vi "SMSMagnet.Contents.vi"   [LabVIEW 2014, in "SMSMagnet.lvlib"]
doc: "This is the constructor of a class.\n\nLicense Agreement for this software:\n\nCopyright (C)\nGesellschaft für Schwerionenforschung, GSI\nPlanckstr. 1\n64291 Darmstadt\nGermany\n\nContact: D.Beck@gsi.de \n\nThis program is free software; you can redistribute it and/or modify it under the terms of the \nGNU General Public License as published by the Free Software Foundation; either version 2 of \nthe license, or (at your option) any later version.\n\nThis program is distributed in the hope that it will be useful, but WITHOUT ANY WARRANTY; \nwithout even the implied warranty of MERCHANTABILITY or FITNESS FOR A PARTICULAR PURPOSE. See the GNU General License for more details (http://www.gnu.org).\n\nGesellschaft für Schwerionenforschung, GSI\nPlanckstr. 1, 64291 Darmstadt, Germany\nFor all questions and ideas contact: M.Richter@gsi.de, H.Brand@gsi.de or D.Beck@gsi.de.\nLast update: 16-JUN-2004"
uses:
  SMSMagnet.lvlib
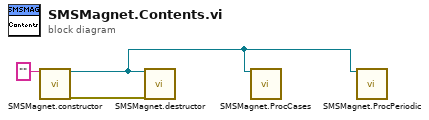
[diagram p0: block diagram]
diagram:
  n1 = call "SMSMagnet.constructor.vi"("name"="") -> ("i ref out"=w1:refnum<vi>, "error out"=w3:errorcluster)  [unwired: 16 in, 1 out]
  n2 = call "SMSMagnet.destructor.vi"("i ref in"=w1, "error in (no error)"=w3) -> ()  [unwired: 17 in, 1 out]
  n3 = call "SMSMagnet.ProcCases.vi"("i ref in"=w1) -> ()  [unwired: 16 in, 3 out]
  n4 = call "SMSMagnet.ProcPeriodic.vi"("i ref in"=w1) -> ()  [unwired: 16 in, 3 out]
